vi "set_written_to_device.vi"(8 "error in (no error)":errorcluster, 10 "written to device?":bool, 11 "DAQmxWriteSignals in":refnum<class "SignalWriterMM140725DAQmx.lvclass">) -> (0 "error out":errorcluster, 3 "DAQmxWriteSignals out":refnum<class "SignalWriterMM140725DAQmx.lvclass">)   [LabVIEW 2010, in "SignalWriterMM140725DAQmx.lvclass"]
uses:
  SignalWriterMM140725DAQmx.lvclass
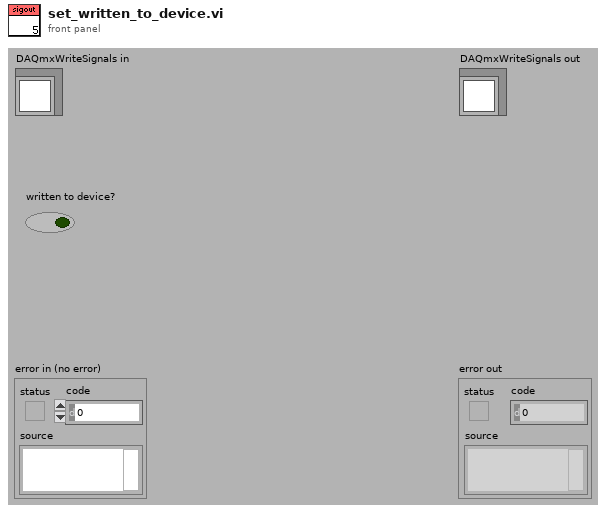
[diagram p1: front panel]
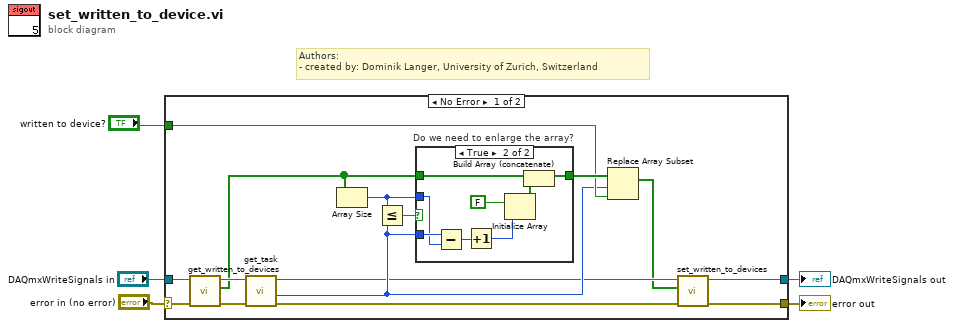
[diagram p0: block diagram]
diagram:
  # "Authors: \n- created by: Dominik Langer, University of Zurich, Switzerland"
  n1 = case shown="No Error" "error in (no error)" {
    selector: "error in (no error)" -> [w15 w31]
    tunnel: [w10 w31] -> w4
    tunnel: [w7 w30] -> w2
    tunnel: "DAQmxWriteSignals in" -> [w12 w30]
    tunnel: "written to device?" -> [w18 _]
    frame No Error {
      n2 = call-dynamic "get_written_to_devices.vi"("error in (no error)"=w15, "DAQmxWriteSignals in"=w12) -> ("error out"=w14:errorcluster, "written to devices?"=w11:bool[], "DAQmxWriteSignals out"=w13:refnum<class "SignalWriterMM140725DAQmx.lvclass">)  [unwired: 7 out]
      n3 = call-dynamic "get_task.vi"("error in (no error)"=w14, "DAQmxWriteSignals in"=w13) -> ("error out"=w9:errorcluster, "index"=w16:i32, "DAQmxWriteSignals out"=w8:refnum<class "SignalWriterMM140725DAQmx.lvclass">)  [unwired: 7 out]
      n4 = Array Size(array=w11) -> (size(s)=w17:i32)
      n5 = Less Or Equal?(x=w17, y=w16) -> (x <= y?=w20:bool)
      n6 = case "Do we need to enlarge the array?" shown="True" w20 {
        tunnel: [w21 w28] -> w19
        tunnel: w11 -> [w21 w29]
        tunnel: w17 -> [_ w24]
        tunnel: w16 -> [_ w25]
        frame False {
        }
        frame True {
          n7 = Subtract(x=w25, y=w24) -> (x-y=w23:i32)
          n8 = Increment(x=w23) -> (x+1=w22:i32)
          n9 = Initialize Array(FALSE, w22) -> (w26:bool[])
          n10 = Build Array (concatenate)(w29, w26) -> (w28:bool[])
        }
      }
      n11 = Replace Array Subset(array=w19, new element=w18, index=w16) -> (w6:bool[])
      n12 = call-dynamic "set_written_to_devices.vi"("error in (no error)"=w9, "written to devices?"=w6, "DAQmxWriteSignals in"=w8) -> ("error out"=w10:errorcluster, "DAQmxWriteSignals out"=w7:refnum<class "SignalWriterMM140725DAQmx.lvclass">)  [unwired: 7 out]
    }
    frame Error {
    }
  }
  "error out" <- w4
  "DAQmxWriteSignals out" <- w2
